vi "Read Config File.vi"(8 "error in (no error)":errorcluster, 10 "create file if necessary? (F)":bool, 11 "appended path":path) -> (0 "error out":errorcluster, 1 "Data":cluster{"Keys":string[], "Values":string[]}[](array[cluster]), 2 "section names":string[](array[string]), 3 "Alt Data":T1(array[cluster]), 4 "File Exists?":bool)   [LabVIEW 2017]
uses:
  <vilib>/Utility/config.llb/Read Key (String).vi
  <vilib>/Utility/config.llb/NI_LVConfig.lvlib
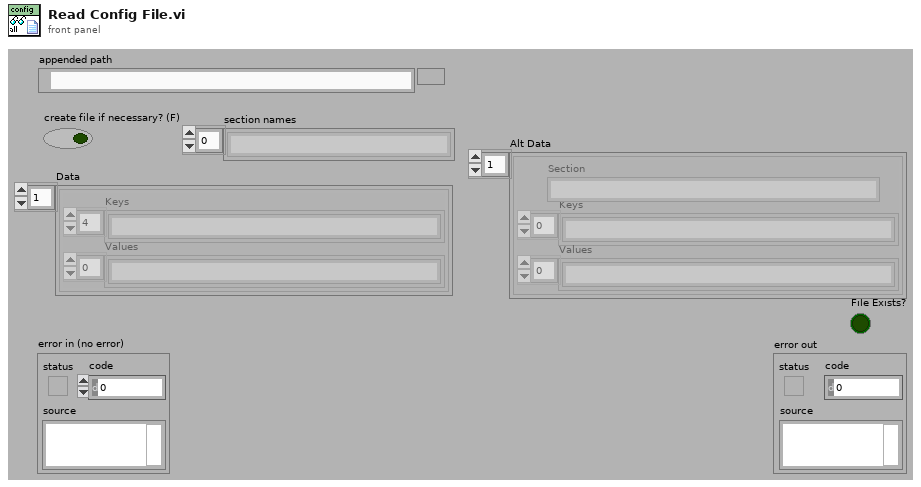
[diagram p1: front panel]
types:
  T1 = cluster{"Section":string, "Keys":string[], "Values":string[]}[]
  T2 = typedef "NI_LVConfig.lvlib/Config Data RefNum.ctl" = refnum<k1>
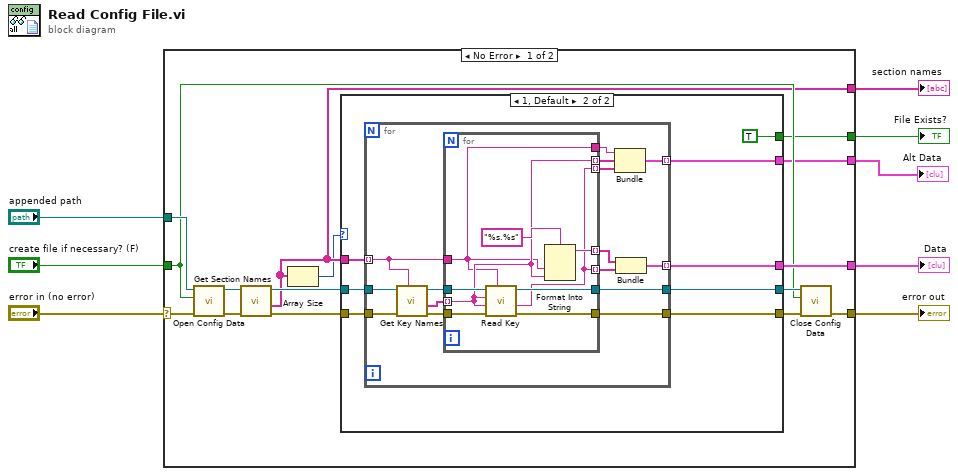
[diagram p0: block diagram]
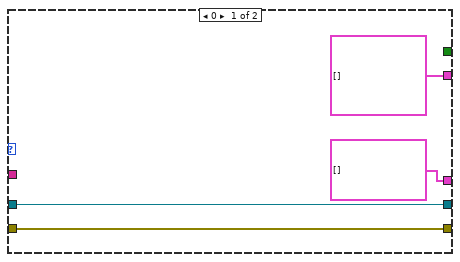
[diagram p2: hidden frame]
diagram:
  n1 = case shown="No Error" "error in (no error)" {
    selector: "error in (no error)" -> [w14 w60]
    tunnel: "appended path" -> [w23 _]
    tunnel: [w12 _] -> w7
    tunnel: [w22 _] -> w6
    tunnel: [w21 w60] -> w5
    tunnel: "create file if necessary? (F)" -> [w13 _]
    tunnel: [w10 _] -> w2
    tunnel: [w9 _] -> w1
    frame No Error {
      n2 = call <vilib>:"Open Config Data.vi"("error in (no error)"=w14, "create file if necessary (T)"=w13, "configuration file path"=w23) -> ("error out"=w20:errorcluster, "refnum"=w19:T2)  [unwired: 6 in, 1 out]
      n3 = call <vilib>:"Get Section Names.vi"("error in (no error)"=w20, "refnum"=w19) -> ("error out"=w18:errorcluster, "section names"=w12:string[], "refnum out"=w17:T2)  [unwired: 7 in]
      n4 = Array Size(array=w12) -> (size(s)=w11:i32)
      n5 = case shown="1, Default" w11 {
        tunnel: w12 -> [_ w35]
        tunnel: [cluster{string[], string[]}[] [] w34] -> w22
        tunnel: w18 -> [w27 w33]
        tunnel: w17 -> [w26 w32]
        tunnel: [w26 w31] -> w16
        tunnel: [w27 w30] -> w15
        tunnel: [_ TRUE] -> w10
        tunnel: [cluster{"String":string, string[], string[]}[] [] w28] -> w9
        frame 0 {
        }
        frame 1, Default {
          n6 = for {
            tunnel: w33 -> [w50]
            tunnel: w32 -> [w49]
            tunnel: w35 -> [w46] mode=indexing
            tunnel: [w45] -> w31
            tunnel: [w44] -> w30
            tunnel: [w40] -> w34 mode=indexing
            tunnel: [w36] -> w28 mode=indexing
            n7 = call <vilib>:"Get Key Names.vi"("section"=w46, "error in (no error)"=w50, "refnum"=w49) -> ("error out"=w47:errorcluster, "key names"=w43:string[], "refnum out"=w48:T2)  [unwired: 5 in, 1 out]
            n8 = for {
              tunnel: w48 -> [w59]
              tunnel: w43 -> [w53] mode=indexing
              tunnel: [w52] -> w41 mode=indexing
              tunnel: [w58] -> w45
              tunnel: w47 -> [w57]
              tunnel: [w56] -> w44
              tunnel: w46 -> [w51]
              tunnel: [w54] -> w42 mode=indexing
              tunnel: [w53] -> w39 mode=indexing
              tunnel: [w52] -> w38 mode=indexing
              tunnel: [w51] -> w37
              n9 = call-poly <vilib>:"Read Key.vi"("section"=w51, "error in (no error)"=w57, "default value"=w53, "key"=w53, "refnum"=w59) -> ("error out"=w56:errorcluster, "value"=w52:string, "refnum out"=w58:T2)  [unwired: 3 in, 1 out]
              n10 = Format Into String(format string="%s.%s", w51, w53) -> (resulting string=w54:string)  [unwired: 2 in, 1 out]
            }
            n11 = Bundle("String"=w37, w39, w38) -> (w36:cluster{"String":string, string[], string[]})  [unwired: 1 in]
            n12 = Bundle(w42, w41) -> (w40:cluster{string[], string[]})  [unwired: 1 in]
          }
        }
      }
      n13 = call <vilib>:"Close Config Data.vi"("error in (no error)"=w15, "write file if changed (T)"=w13, "refnum"=w16) -> ("error out"=w21:errorcluster)  [unwired: 7 in, 1 out]
    }
    frame Error {
    }
  }
  "section names" <- w7
  "Data" <- w6
  "error out" <- w5
  "File Exists?" <- w2
  "Alt Data" <- w1
